vi "Drop Down VI Loader.vi"(7 "Software Config File Path":path=path "C:/Users/Ries Lab/Documents/Microscope Control from Sheng Account/Microscope-Control/Drop Down VI Loader/Drop Down VI Loader Config Files/EMBL 4Pi.txt") -> ()   [LabVIEW 2021]
uses:
  Drop Down VI Loader Type Defs/DDVL Drop Down Bar.ctl
  <vilib>/Utility/miscctls.llb/LVPointTypeDef.ctl
  <vilib>/Utility/miscctls.llb/LVRectTypeDef.ctl
panel:
  in  "Drop Down Control 20":T1
  in  "Drop Down Control 19":T1
  in  "Drop Down Control 18":T1
  in  "Drop Down Control 17":T1
  in  "Drop Down Control 16":T1
  in  "Drop Down Control 15":T1
  in  "Drop Down Control 14":T1
  in  "Drop Down Control 13":T1
  in  "Drop Down Control 12":T1
  in  "Drop Down Control 11":T1
  in  "Hide Exit Bar":bool
  in  "Hide Drop Bars":bool
  in  "Screen and Exit Bar":T2
  in  "Drop Down Control 01":T1
  in  "Drop Down Control 02":T1
  in  "Drop Down Control 03":T1
  in  "Drop Down Control 04":T1
  in  "Drop Down Control 05":T1
  in  "Drop Down Control 06":T1
  in  "Drop Down Control 07":T1
  in  "Drop Down Control 08":T1
  in  "Drop Down Control 09":T1
  in  "Drop Down Control 10":T1
  # "Some Text"
  # "Some Text"
  # "Some Text"
  # "Some Text"
  # "Some Text"
  # "Some Text"
  # "Some Text"
  # "Some Text"
  # "Some Text"
  # "Some Text"
  # "Blank 01"
  # "Blank 02"
  # "Blank 03"
  # "Blank 04"
  # "Blank 05"
  # "Blank 06"
  # "Blank 07"
  # "Blank 08"
  # "Some Text"
  # "Some Text"
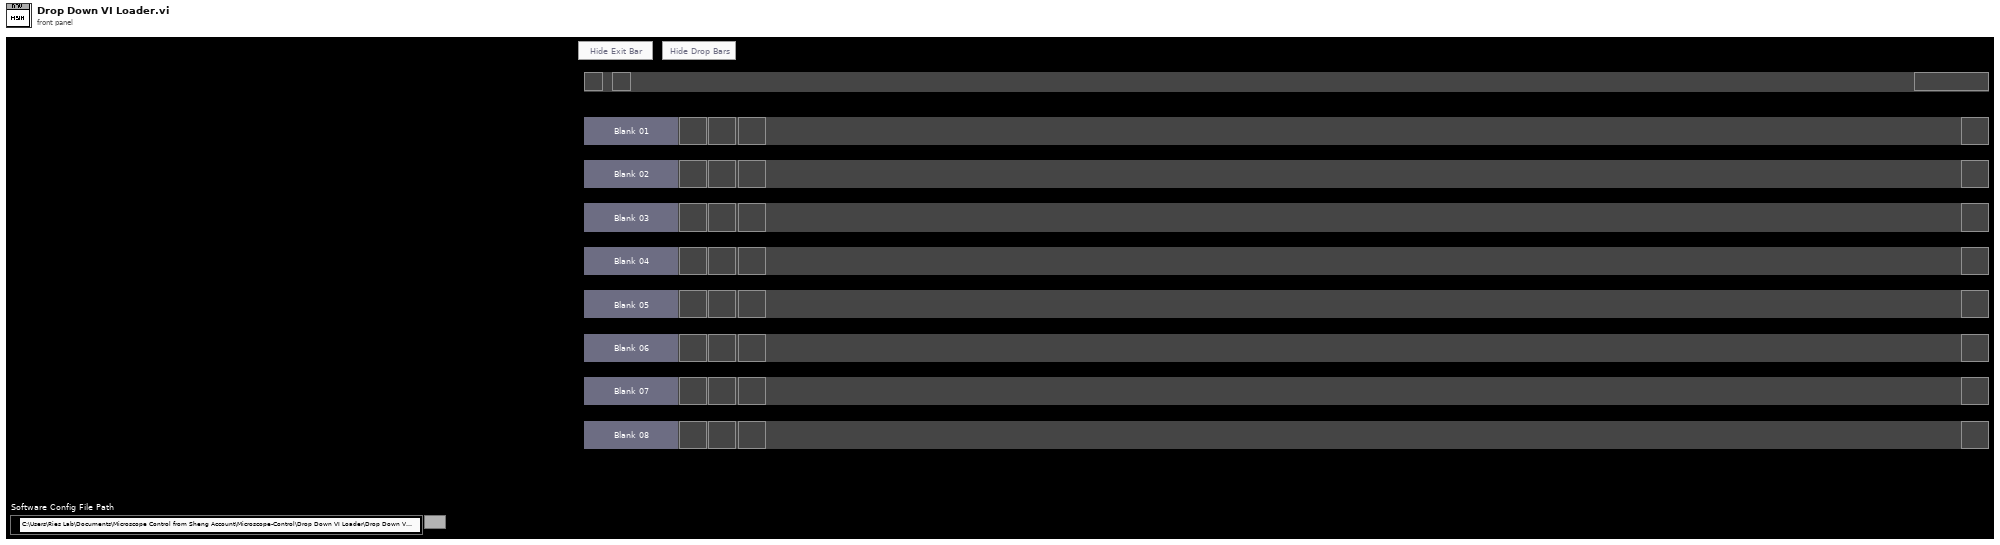
[diagram p1: front panel]
types:
  T1 = typedef "DDVL Drop Down Bar.ctl" = cluster{"Right Width":bool, "Messages":string, "Abort VI":bool, "Close VI":bool, "Pop Out":bool}
  T2 = cluster{"Max Left":bool, "Max Right":bool, "Exit":bool, "Messages":string}
  T3 = enum16{"Always On", "Always Off", "Off While Running"}
  T4 = typedef "LVPointTypeDef.ctl" = cluster{"Horizontal":i16, "Vertical":i16}
  T5 = enum32{"Invalid", "Standard", "Closed", "Hidden", "Minimized", "Maximized"}
  T6 = typedef "LVRectTypeDef.ctl" = cluster{"Left":i16, "Top":i16, "Right":i16, "Bottom":i16}
  T7 = enum8{"Enabled", "Disabled", "Disabled and Grayed Out"}
  T8 = cluster{"VI Path":path, "VI Refnum":refnum<vi>}[]
  T9 = typedef "lveventtype.ctl" = enum32{"Null", "Timeout", "Annotation Menu Selection", "Annotation Menu Selection?", "App Instance Close", "App Instance Close?", "Autoscale Range Change", "Bookmark Info Change", "Cell Edit", "Cell Edit?", "Cursor Grab", "Cursor Grab?", "Cursor Menu Selection", "Cursor Menu Selection?", "Cursor Move", "Cursor Release", "Data Change", "Direction Change", "Display State Change", "Drag Ended", "Drag Enter", "Drag Leave", "Drag Over", "Drag Source Update", "Drag Starting", "Drag Starting?", "Drop", "Exec State Change", "Key Down", "Key Down?", "Key Repeat", "Key Repeat?", "Key Up", "Listbox Double Click", "Menu Activation?", "Menu Selection (App)", "Menu Selection? (App)", "Menu Selection (User)", "Mouse Down", "Mouse Down?", "Mouse Enter", "Mouse Leave", "Mouse Move", "Mouse Up", "Mouse Wheel", "NI Security User Change (App)", "Pane Size", "Panel Close", "Panel Close?", "Panel Resize", "Plot Attribute Change", "Scale Range Change", "Shortcut Menu Activation?", "Shortcut Menu Selection (App)", "Shortcut Menu Selection? (App)", "Shortcut Menu Selection (User)", "Tree Double Click", "Tree Drag", "Tree Drag?", "Tree Drop", "Tree Drop?", "Tree Item Close", "Tree Item Close?", "Tree Item Open", "Tree Item Open?", "User Event", "Value Change"}
  T10 = typedef "LVAllMonitorsDisplayTypeDef.ctl" = cluster{"Bounds":cluster{"Left":i16, "Top":i16, "Right":i16, "Bottom":i16}, "Depth":i16}[]
  T11 = cluster{"Bounds":cluster{"Left":i16, "Top":i16, "Right":i16, "Bottom":i16}, "Depth":i16}
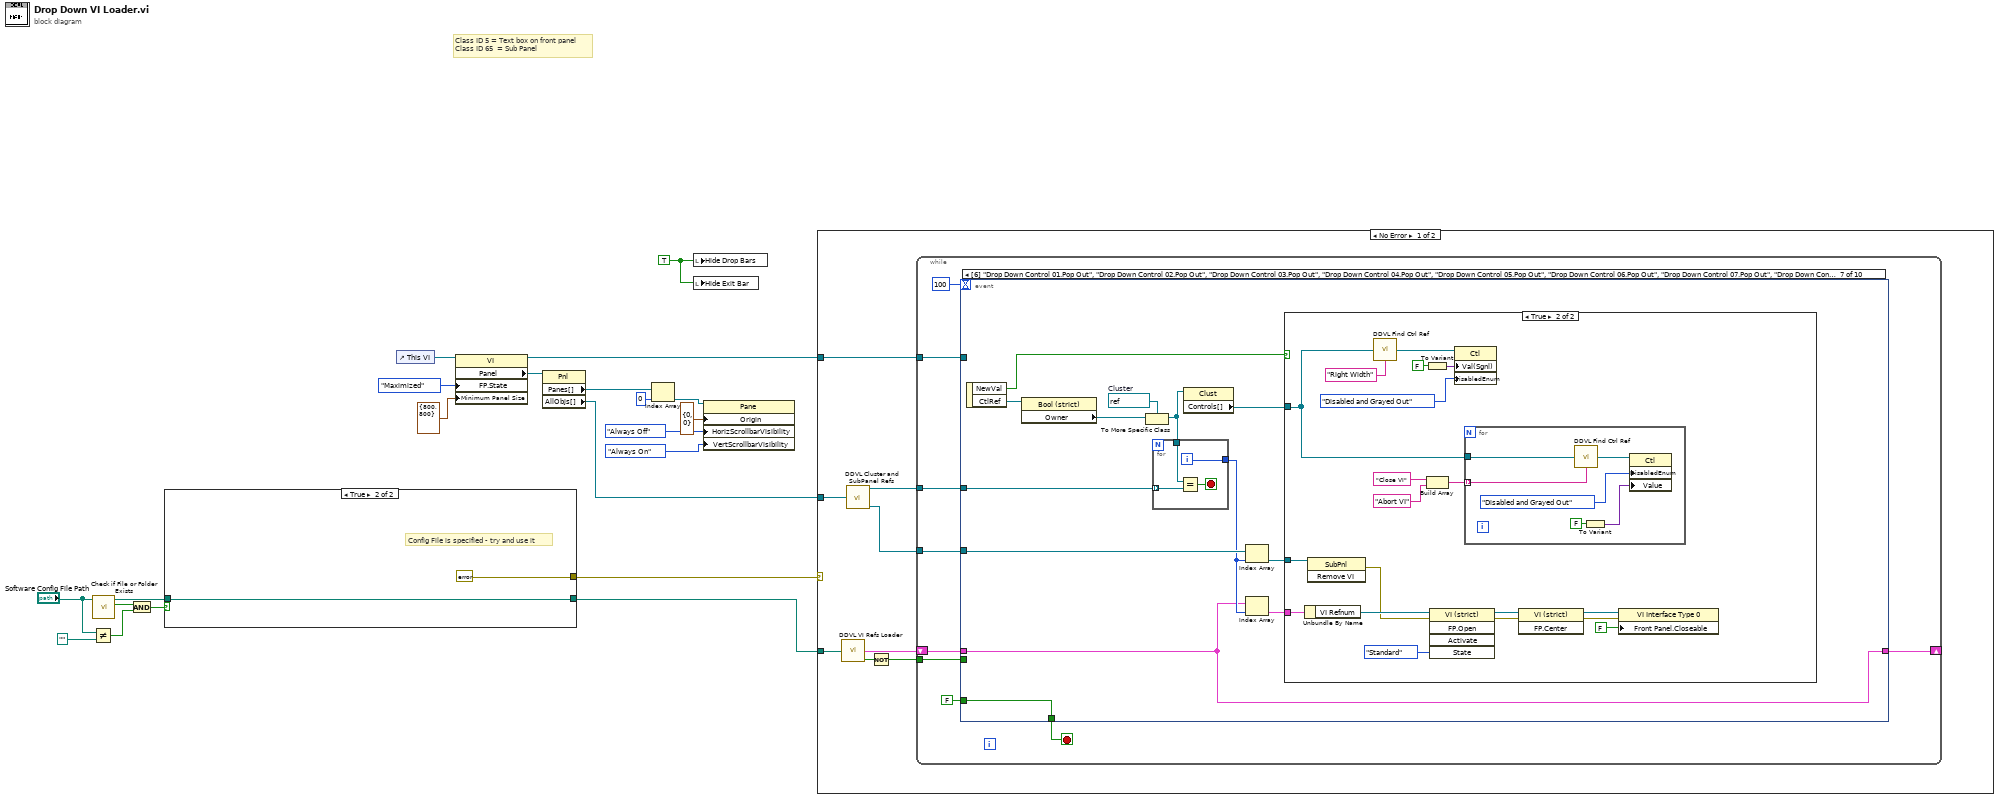
[diagram p0: block diagram]
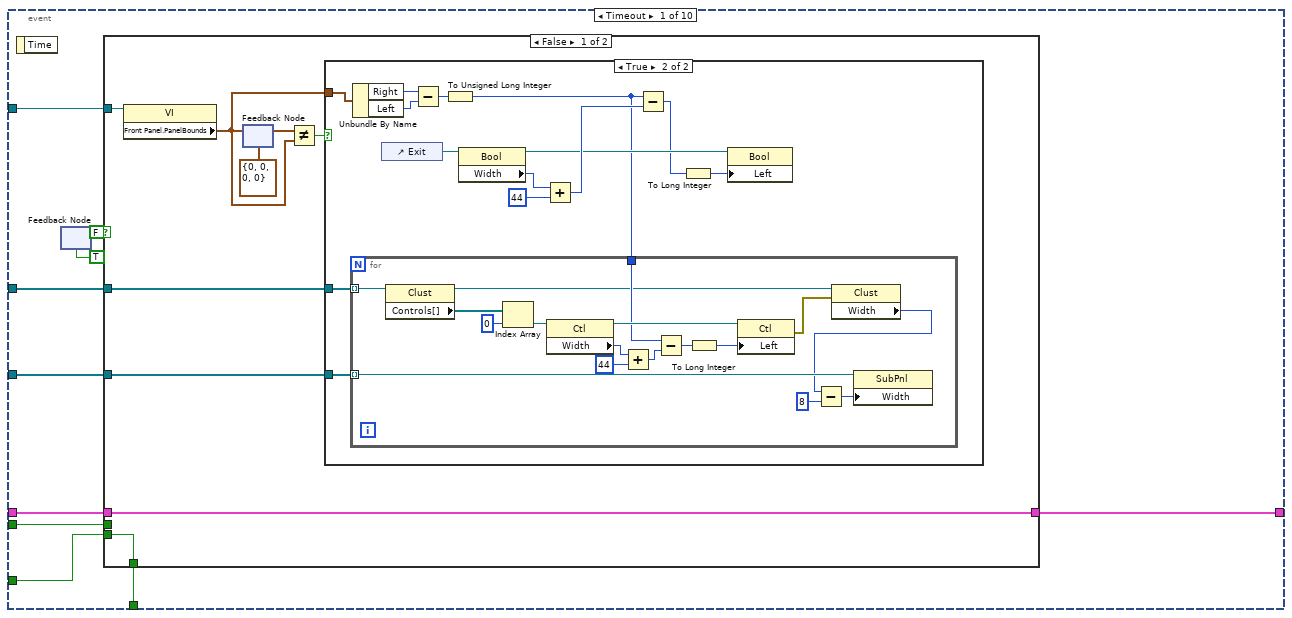
[diagram p2: hidden frame]
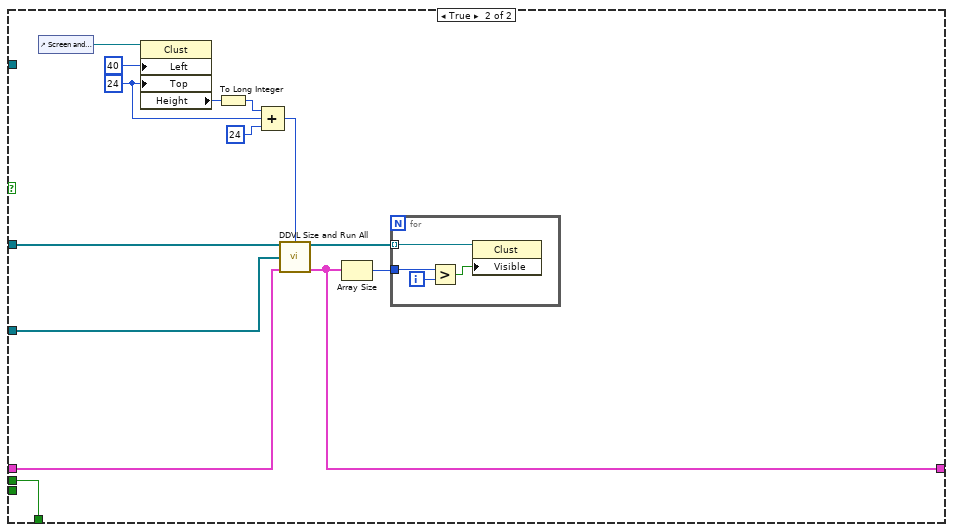
[diagram p4: hidden frame]
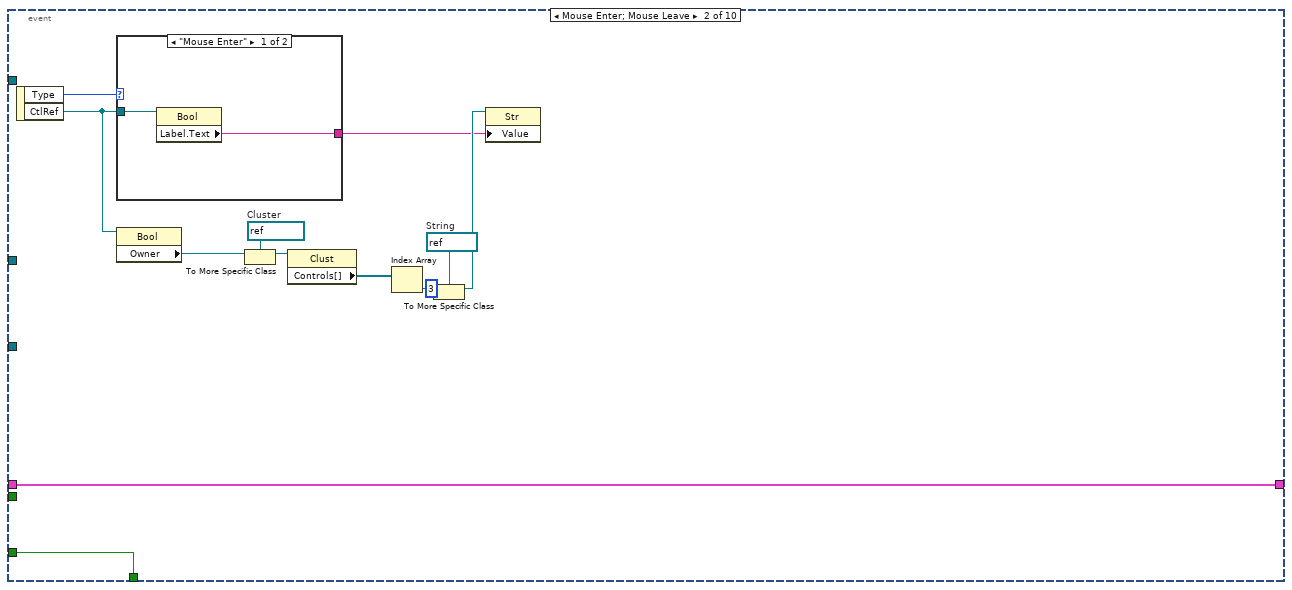
[diagram p5: hidden frame]
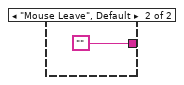
[diagram p6: hidden frame]
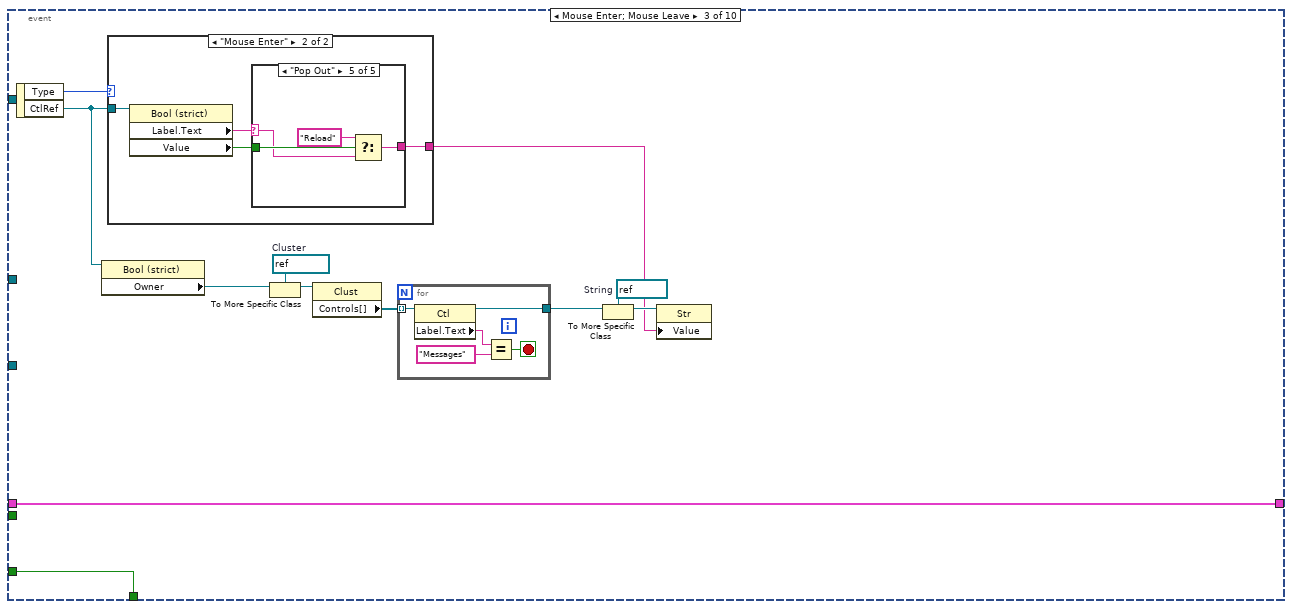
[diagram p7: hidden frame]
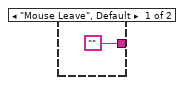
[diagram p8: hidden frame]
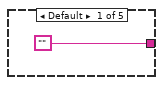
[diagram p9: hidden frame]
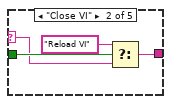
[diagram p10: hidden frame]
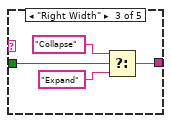
[diagram p11: hidden frame]
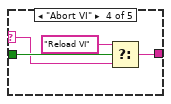
[diagram p12: hidden frame]
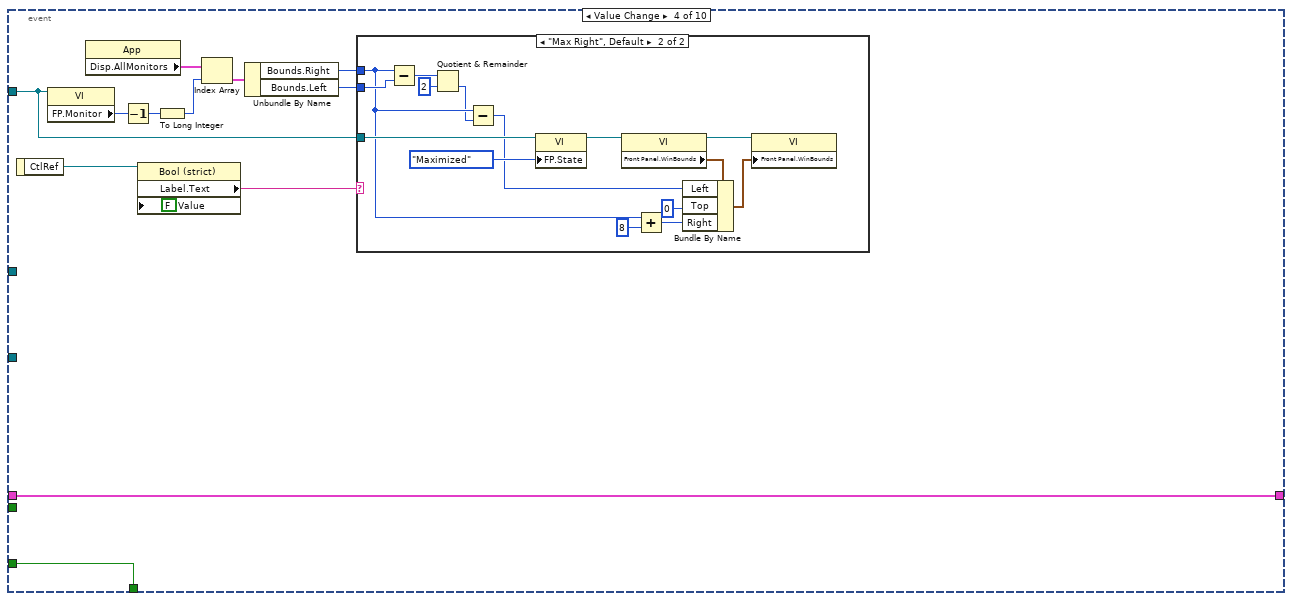
[diagram p13: hidden frame]
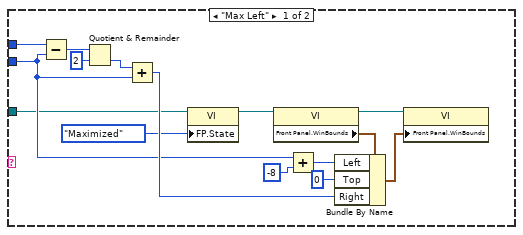
[diagram p14: hidden frame]
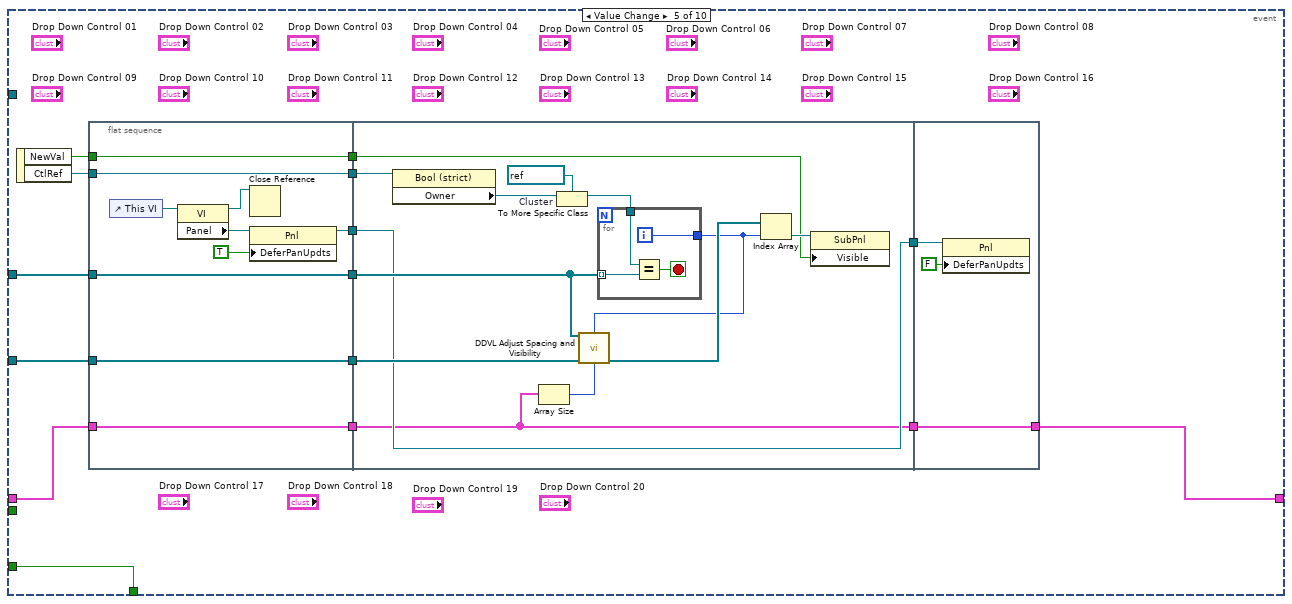
[diagram p15: hidden frame]
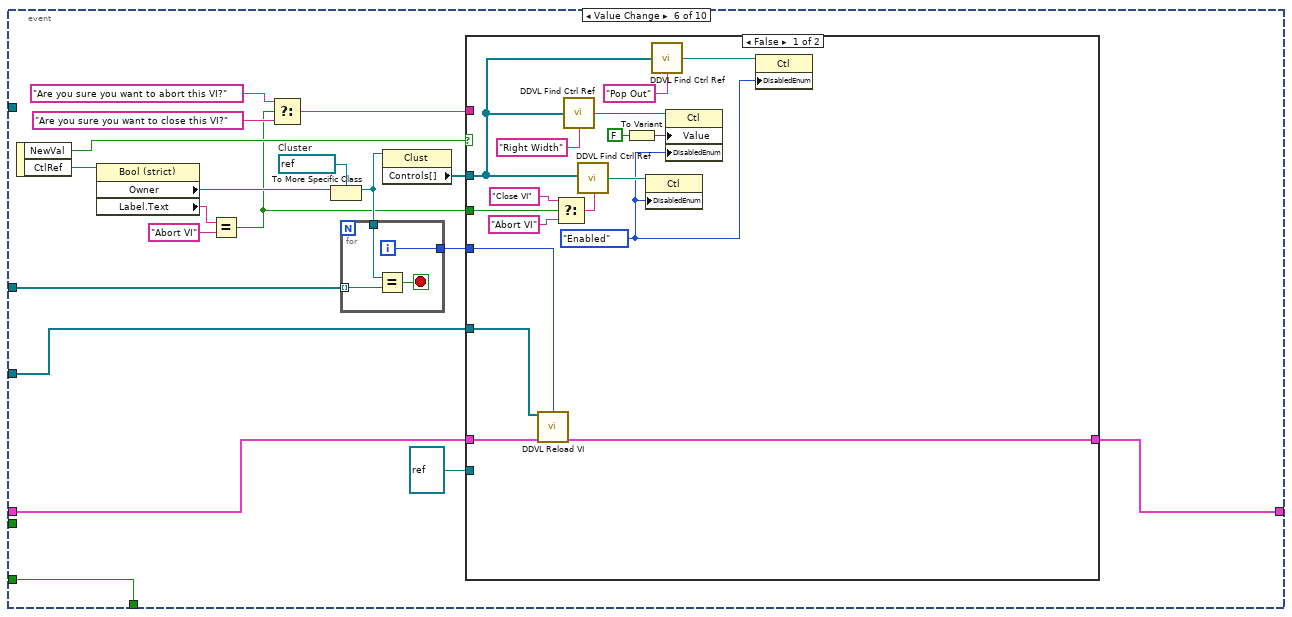
[diagram p16: hidden frame]
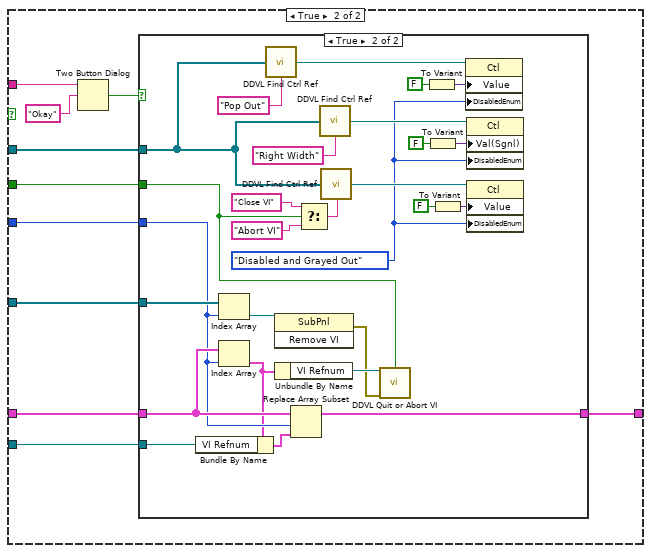
[diagram p17: hidden frame]
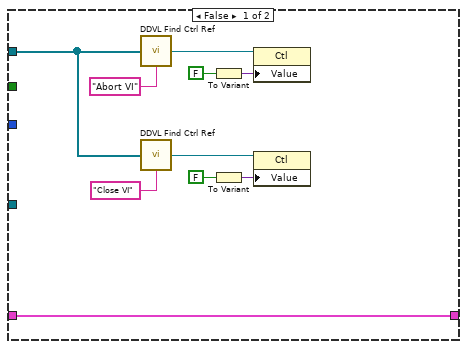
[diagram p18: hidden frame]
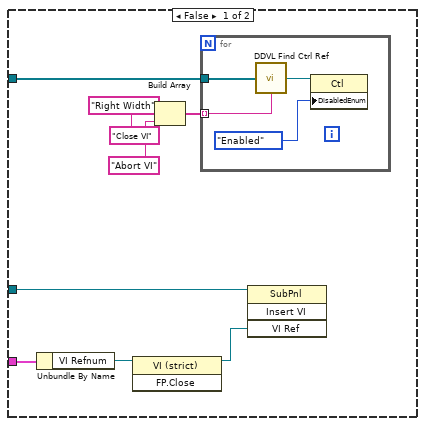
[diagram p19: hidden frame]
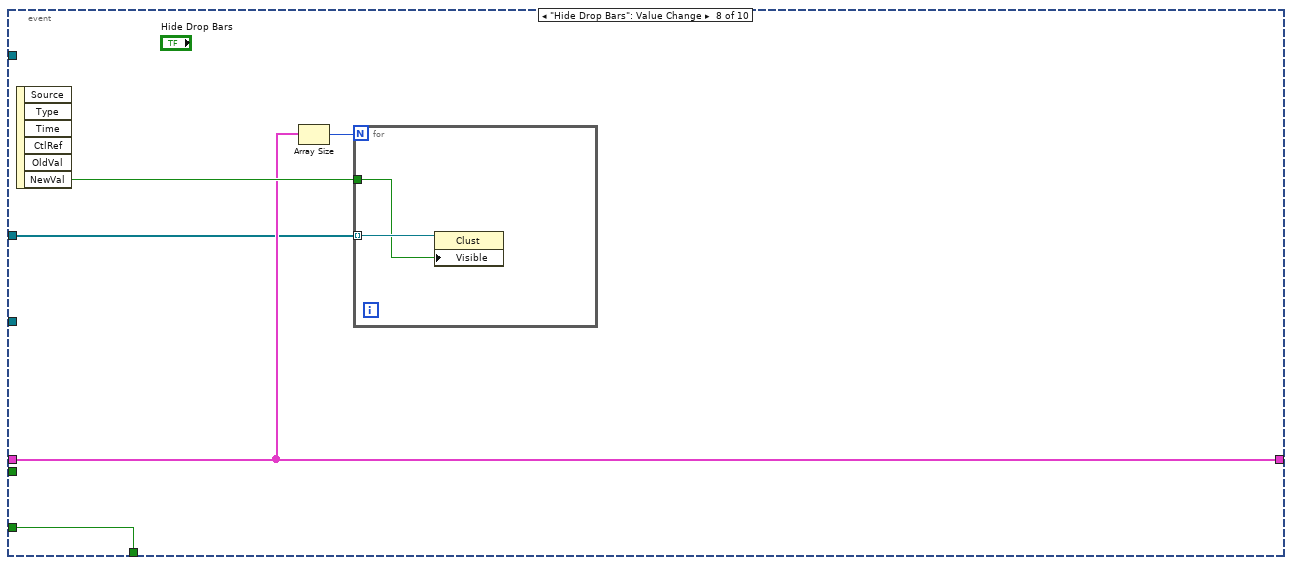
[diagram p20: hidden frame]
diagram:
  w1 = TRUE ("Hide Drop Bars")
  # "Class ID 5 = Text box on front panel\nClass ID 65  = Sub Panel"
  n1 = Not Equal?(x="Software Config File Path", y=path "") -> (x != y?=w8:bool)
  n2 = call <vilib>:"Check if File or Folder Exists.vi"("path"="Software Config File Path") -> ("file or folder exists?"=w7:bool, "dup path"=w5:path)  [unwired: 8 in, 1 out]
  n3 = And(x=w7, y=w8) -> (x .and. y?=w6:bool)
  n4 = case shown="True" w6 {
    tunnel: w5 -> [_ w34]
    tunnel: [w30 w34] -> w2
    tunnel: [w29 errorcluster {"status"=FALSE, "code"=0, "source"=""} ("error out")] -> w3
    frame False {
      # "User must select config file"
      n5 = control-ref of="This VI"() -> (w24:refnum<vi>)
      n6 = property class="VI"(reference=w24) -> ("Path"=w23:path)  [unwired: 1 in, 2 out]
      n7 = Strip Path(path=w23) -> (stripped path=w25:path)  [unwired: 1 out]
      n8 = Path To String(path=w25) -> (string=w26:string)
      n9 = Concatenate Strings(w26, "\\Drop Down VI Loader Config Files") -> (w28:string)
      n10 = String To Path(string=w28) -> (path=w22:path)
      n11 = call "File Dialog"("start path"=w22, "prompt"="Select Software Config File", "pattern (all files)"="*.txt") -> ("selected path"=w30:path, "error out"=w29:errorcluster)  [unwired: 9 in, 2 out]
    }
    frame True {
      # "Config File is specified - try and use it"
    }
  }
  n12 = control-ref of="This VI"() -> (w17:refnum<vi>)
  n13 = property class="VI"(reference=w17, "FP.State"=T5."Maximized" ("Front Panel Window:State"), "Minimum Panel Size"=T4 {"Horizontal"=800, "Vertical"=800} ("Front Panel Window:Minimum Size")) -> (reference out=w12:refnum<vi>, "Panel"=w11:refnum<vi>)  [unwired: 1 in, 1 out]
  n14 = property class="Pnl"(reference=w11) -> ("Panes[]"=w14:refnum<vi>[], "AllObjs[]"=w10:refnum<vi>[])  [unwired: 1 in, 2 out]
  n15 = Index Array(array=w14, index=0) -> (element=w20:refnum<vi>)
  n16 = local write "Hide Drop Bars"(w1) -> ()
  n17 = local write "Hide Exit Bar"(w1) -> ()
  n18 = property class="Pane"(reference=w20, "Origin"=T4 {"Horizontal"=0, "Vertical"=0}, "HorizScrollbarVisibility"=T3."Always Off" ("Vertical Scrollbar Visibility"), "VertScrollbarVisibility"=T3."Always On" ("Vertical Scrollbar Visibility")) -> ()  [unwired: 1 in, 2 out]
  n19 = case shown="No Error" w3 {
    tunnel: w12 -> [w42 _]
    tunnel: w10 -> [w40 _]
    tunnel: w2 -> [w37 _]
    frame No Error {
      n20 = call "DDVL VI Refs Loader.vi"("Config File Path"=w37) -> ("VI Path/Ref"=w39:T8, "VIs Loaded?"=w41:bool)  [unwired: 12 in, 1 out]
      n21 = call "DDVL Cluster and SubPanel Refs.vi"("All Objects Refs"=w40) -> ("Cluster Refs"=w36:refnum<vi>[], "Sub Panel Refs"=w35:refnum<vi>[])  [unwired: 13 in]
      n22 = Not(x=w41) -> (.not. x?=w38:bool)
      n23 = while {
        tunnel: w42 -> [w48]
        tunnel: w36 -> [w43]
        tunnel: w35 -> [w46]
        tunnel: w38 -> [w45]
        shift-right: [w44] -> _
        shift-left: w39 -> [w47]
        stop <- w51 stop-if-true
        n24 = event shown="[6] \"Drop Down Control 01.Pop Out\", \"Drop Down Control 02.Pop Out\", \"Drop Down Control 03.Pop Out\", \"Drop Down Control 04.Pop Out\", \"Drop Down Control 05.Pop Out\", \"Drop Down Control 06.Pop Out\", \"Drop Down Control 07.Pop Out\", \"Drop Down Control 08.Pop Out\", \"Drop Down Control 09.Pop Out\", \"Drop Down Control 10.Pop Out\", \"Drop Down Control 11.Pop Out\", \"Drop Down Control 12.Pop Out\", \"Drop Down Control 13.Pop Out\", \"Drop Down Control 14.Pop Out\", \"Drop Down Control 15.Pop Out\", \"Drop Down Control 16.Pop Out\", \"Drop Down Control 17.Pop Out\", \"Drop Down Control 18.Pop Out\", \"Drop Down Control 19.Pop Out\", \"Drop Down Control 20.Pop Out\": Value Change" {
          selector: _ -> [_ _ _ _ _ _ _ _ _ _]
          dyn-events: _ -> [_ _ _ _ _ _ _ _ _ _]
          timeout: 100 -> [_ _ _ _ _ _ _ _ _ _]
          tunnel: [w58 w133 w147 w188 w233 w282 w363 w410 w416 w432] -> w51
          tunnel: FALSE -> [w57 w133 w147 w188 w233 w282 w363 w410 w416 _]
          tunnel: w48 -> [w62 _ _ w179 _ _ _ _ _ _]
          tunnel: w43 -> [w61 _ _ _ w231 w277 w357 w406 _ w430]
          tunnel: w46 -> [w60 _ _ _ w232 w275 w356 _ _ w429]
          tunnel: w47 -> [w59 w121 w148 w176 w228 w276 w352 w407 w415 w428]
          tunnel: w45 -> [w56 _ _ _ _ _ _ _ _ _]
          tunnel: [w55 w121 w148 w176 w220 w273 w352 w407 w415 w427] -> w44
          event Timeout {
            n25 = event-data() -> ()  [unwired: 1 in, 1 out]
            n26 = feedback #1(TRUE) -> (w52:bool)
            n27 = feedback-in #1(FALSE) -> ()
            n28 = case shown="False" w52 {
              tunnel: w62 -> [w71 _]
              tunnel: w61 -> [w66 w107]
              tunnel: w60 -> [w65 w114]
              tunnel: w59 -> [w63 w113]
              tunnel: [w64 w104] -> w58
              tunnel: w57 -> [w64 _]
              tunnel: w56 -> [_ w104]
              tunnel: [w63 w103] -> w55
              frame False {
                n29 = property class="VI"(reference=w71) -> ("Front Panel.PanelBounds"=w67:T6)  [unwired: 1 in, 2 out]
                n30 = feedback-in #2(w67) -> ()
                n31 = feedback #2(T6 {"Left"=0, "Top"=0, "Right"=0, "Bottom"=0} ("Front Panel.PanelBounds")) -> (w70:T6)
                n32 = Not Equal?(x=w70, y=w67) -> (x != y?=w68:bool)
                n33 = case shown="True" w68 {
                  tunnel: w67 -> [_ w85]
                  tunnel: w66 -> [_ w75]
                  tunnel: w65 -> [_ w72]
                  frame False {
                  }
                  frame True {
                    n34 = Unbundle By Name(w85) -> ("Right"=w77:i16, "Left"=w78:i16)
                    n35 = control-ref of="Exit"() -> (w83:refnum<vi>)
                    n36 = Subtract(x=w77, y=w78) -> (x-y=w76:i16)
                    n37 = To Unsigned Long Integer(number=w76) -> (unsigned 32bit integer=w73:u32)
                    n38 = for {
                      tunnel: w75 -> [w102] mode=indexing
                      tunnel: w73 -> [w93]
                      tunnel: w72 -> [w91] mode=indexing
                      n39 = property class="Clust"(reference=w102) -> (reference out=w90:refnum<vi>, "Controls[]"=w101:refnum<vi>[])  [unwired: 1 in, 1 out]
                      n40 = Index Array(array=w101, index=0) -> (element=w97:refnum<vi>)
                      n41 = property class="Ctl"(reference=w97) -> (reference out=w96:refnum<vi>, "Width"=w98:u32)  [unwired: 1 in, 1 out]
                      n42 = Add(x=w98, y=u32 44) -> (x+y=w95:u32)
                      n43 = Subtract(x=w93, y=w95) -> (x-y=w94:u32)
                      n44 = To Long Integer(number=w94) -> (32bit integer=w99:i32)
                      n45 = property class="Ctl"(reference=w96, "Left"=w99) -> (error out=w89:errorcluster)  [unwired: 1 in, 1 out]
                      n46 = property class="Clust"(reference=w90, error in=w89) -> ("Width"=w88:u32)  [unwired: 2 out]
                      n47 = Subtract(x=w88, y=u32 8) -> (x-y=w87:u32)
                      n48 = property class="SubPnl"(reference=w91, "Width"=w87) -> ()  [unwired: 1 in, 2 out]
                    }
                    n49 = property class="Bool"(reference=w83) -> (reference out=w81:refnum<vi>, "Width"=w84:u32)  [unwired: 1 in, 1 out]
                    n50 = Add(x=w84, y=u32 44) -> (x+y=w82:u32)
                    n51 = Subtract(x=w73, y=w82) -> (x-y=w79:u32)
                    n52 = To Long Integer(number=w79) -> (32bit integer=w80:i32)
                    n53 = property class="Bool"(reference=w81, "Left"=w80) -> ()  [unwired: 1 in, 2 out]
                  }
                }
              }
              frame True {
                w111 = 24 ("Position:Top")
                n54 = control-ref of="Screen and Exit Bar"() -> (w116:refnum<vi>)
                n55 = property class="Clust"(reference=w116, "Left"=40 ("Position:Left"), "Top"=w111) -> ("Height"=w112:u32)  [unwired: 1 in, 2 out]
                n56 = To Long Integer(number=w112) -> (32bit integer=w110:i32)
                n57 = Compound Arithmetic op=ADD(w110, w111, 24 ("value")) -> (w108:i32)
                n58 = call "DDVL Size and Run All.vi"("Cluster Refs"=w107, "Initial Top Position"=w108, "Subpanel Refs"=w114, "VI Path/Ref"=w113) -> ("Cluster Refs Dup"=w106:refnum<vi>[], "VI Path/Ref Out"=w103:T8)  [unwired: 10 in]
                n59 = Array Size(array=w103) -> (size(s)=w105:i32)
                n60 = for {
                  tunnel: w106 -> [w120] mode=indexing
                  tunnel: w105 -> [w117]
                  i -> [w119]
                  n61 = Greater?(x=w117, y=w119) -> (0:w118:bool)
                  n62 = property class="Clust"(reference=w120, "Visible"=w118) -> ()  [unwired: 1 in, 2 out]
                }
              }
            }
          }
          event "Screen and Exit Bar.Exit", "Screen and Exit Bar.Max Right", "Screen and Exit Bar.Max Left": Mouse Enter; "Screen and Exit Bar.Exit", "Screen and Exit Bar.Max Right", "Screen and Exit Bar.Max Left": Mouse Leave {
            w124 = refnum<vi> refnum  # String
            w129 = refnum<vi> refnum  # Cluster
            n63 = event-data() -> ("Type"=w132:T9, "CtlRef"=w131:refnum<vi>)  [unwired: 1 in]
            n64 = case shown="\"Mouse Enter\"" w132 {
              tunnel: w131 -> [w135 _]
              tunnel: [w134 ""] -> w122
              frame "Mouse Enter" {
                n65 = property class="Bool"(reference=w135) -> ("Label.Text"=w134:string)  [unwired: 1 in, 2 out]
              }
              frame "Mouse Leave", Default {
              }
            }
            n66 = property class="Bool"(reference=w131) -> ("Owner"=w130:refnum<vi>)  [unwired: 1 in, 2 out]
            n67 = To More Specific Class(target class=w129, reference=w130) -> (specific class reference=w128:refnum<vi>)  [unwired: 1 in, 1 out]
            n68 = property class="Clust"(reference=w128) -> ("Controls[]"=w127:refnum<vi>[])  [unwired: 1 in, 2 out]
            n69 = Index Array(array=w127, index=3) -> (element=w125:refnum<vi>)
            n70 = To More Specific Class(target class=w124, reference=w125) -> (specific class reference=w123:refnum<vi>)  [unwired: 1 in, 1 out]
            n71 = property class="Str"(reference=w123, "Value"=w122) -> ()  [unwired: 1 in, 2 out]
          }
          event Mouse Enter; Mouse Leave {
            w139 = refnum<vi> refnum  # String
            w144 = refnum<vi> refnum  # Cluster
            n72 = event-data() -> ("Type"=w146:T9, "CtlRef"=w145:refnum<vi>)  [unwired: 1 in]
            n73 = property class="Bool (strict)"(reference=w145) -> ("Owner"=w142:refnum<vi>)  [unwired: 1 in, 2 out]
            n74 = case shown="\"Mouse Enter\"" w146 {
              tunnel: w145 -> [_ w158]
              tunnel: ["" w155] -> w137
              frame "Mouse Leave", Default {
              }
              frame "Mouse Enter" {
                n75 = property class="Bool (strict)"(reference=w158) -> ("Label.Text"=w157:string, "Value"=w156:bool)  [unwired: 1 in, 2 out]
                n76 = case shown="\"Pop Out\"" w157 {
                  selector: w157 -> [_ w162 _ w169 w173]
                  tunnel: w156 -> [_ w163 w167 w170 w174]
                  tunnel: ["" w160 w164 w168 w172] -> w155
                  frame Default {
                  }
                  frame "Close VI" {
                    n77 = Select(t="Reload VI", s=w163, f=w162) -> (s? t:f=w160:string)
                  }
                  frame "Right Width" {
                    n78 = Select(t="Collapse", s=w167, f="Expand") -> (s? t:f=w164:string)
                  }
                  frame "Abort VI" {
                    n79 = Select(t="Reload VI", s=w170, f=w169) -> (s? t:f=w168:string)
                  }
                  frame "Pop Out" {
                    n80 = Select(t="Reload", s=w174, f=w173) -> (s? t:f=w172:string)
                  }
                }
              }
            }
            n81 = To More Specific Class(target class=w144, reference=w142) -> (specific class reference=w143:refnum<vi>)  [unwired: 1 in, 1 out]
            n82 = property class="Clust"(reference=w143) -> ("Controls[]"=w141:refnum<vi>[])  [unwired: 1 in, 2 out]
            n83 = for {
              tunnel: w141 -> [w153] mode=indexing
              tunnel: [w149] -> w140
              stop <- w150 stop-if-true
              n84 = property class="Ctl"(reference=w153) -> (reference out=w149:refnum<vi>, "Label.Text"=w152:string)  [unwired: 1 in, 1 out]
              n85 = Equal?(x=w152, y="Messages") -> (x = y?=w150:bool)
            }
            n86 = To More Specific Class(target class=w139, reference=w140) -> (specific class reference=w138:refnum<vi>)  [unwired: 1 in, 1 out]
            n87 = property class="Str"(reference=w138, "Value"=w137) -> ()  [unwired: 1 in, 2 out]
          }
          event "Screen and Exit Bar.Max Right", "Screen and Exit Bar.Max Left": Value Change {
            n88 = event-data() -> ("CtlRef"=w187:refnum<vi>)  [unwired: 1 in]
            n89 = property class="VI"(reference=w179) -> ("FP.Monitor"=w186:u16)  [unwired: 1 in, 2 out]
            n90 = property class="App"() -> ("Disp.AllMonitors"=w185:T10)  [unwired: 2 in, 2 out]
            n91 = Decrement(x=w186) -> (x-1=w184:u16)
            n92 = property class="Bool (strict)"(reference=w187, "Value"=FALSE) -> ("Label.Text"=w178:string)  [unwired: 1 in, 2 out]
            n93 = To Long Integer(number=w184) -> (32bit integer=w183:i32)
            n94 = Index Array(array=w185, index=w183) -> (element=w182:T11)
            n95 = Unbundle By Name(w182) -> ("Bounds.Right"=w181:i16, "Bounds.Left"=w180:i16)
            n96 = case shown="\"Max Right\", Default" w178 {
              tunnel: w181 -> [w203 w206]
              tunnel: w180 -> [w191 w210]
              tunnel: w179 -> [w189 w209]
              frame "Max Left" {
                n97 = Subtract(x=w203, y=w191) -> (x-y=w198:i16)
                n98 = Quotient & Remainder(x=w198, y=i16 2) -> (floor(x/y)=w196:i16)  [unwired: 1 out]
                n99 = Add(x=w196, y=w191) -> (x+y=w195:i16)
                n100 = property class="VI"(reference=w189, "FP.State"=T5."Maximized" ("Front Panel Window:State")) -> (reference out=w193:refnum<vi>)  [unwired: 1 in, 1 out]
                n101 = property class="VI"(reference=w193) -> (reference out=w202:refnum<vi>, "Front Panel.WinBounds"=w200:T6)  [unwired: 1 in, 1 out]
                n102 = Add(x=w191, y=i16 -8 ("Left")) -> (x+y=w190:i16)
                n103 = Bundle By Name(cluster=w200, "Left"=w190, "Top"=i16 0, "Right"=w195) -> (w201:T6)
                n104 = property class="VI"(reference=w202, "Front Panel.WinBounds"=w201) -> ()  [unwired: 1 in, 2 out]
              }
              frame "Max Right", Default {
                n105 = Subtract(x=w206, y=w210) -> (x-y=w215:i16)
                n106 = Quotient & Remainder(x=w215, y=i16 2) -> (floor(x/y)=w205:i16)  [unwired: 1 out]
                n107 = Subtract(x=w206, y=w205) -> (x-y=w204:i16)
                n108 = property class="VI"(reference=w209, "FP.State"=T5."Maximized" ("Front Panel Window:State")) -> (reference out=w212:refnum<vi>)  [unwired: 1 in, 1 out]
                n109 = property class="VI"(reference=w212) -> (reference out=w218:refnum<vi>, "Front Panel.WinBounds"=w216:T6)  [unwired: 1 in, 1 out]
                n110 = Add(x=w206, y=i16 8 ("Left")) -> (x+y=w207:i16)
                n111 = Bundle By Name(cluster=w216, "Left"=w204, "Top"=i16 0, "Right"=w207) -> (w217:T6)
                n112 = property class="VI"(reference=w218, "Front Panel.WinBounds"=w217) -> ()  [unwired: 1 in, 2 out]
              }
            }
          }
          event Value Change {
            n113 = event-data() -> ("NewVal"=w229:bool, "CtlRef"=w230:refnum<vi>)  [unwired: 1 in]
            n114 = flat-sequence {
              tunnel: w228 -> [w239]
              tunnel: w229 -> [w240]
              tunnel: w230 -> [w241]
              tunnel: w231 -> [w242]
              tunnel: w232 -> [w243]
              tunnel: [w243] -> w227
              tunnel: [w242] -> w226
              tunnel: [w241] -> w225
              tunnel: [w240] -> w224
              tunnel: [w239] -> w223
              tunnel: [w234] -> w221
              tunnel: w227 -> [w254]
              tunnel: w226 -> [w253]
              tunnel: w225 -> [w252]
              tunnel: w224 -> [w248]
              tunnel: w223 -> [w244]
              tunnel: [w245] -> w222
              tunnel: w221 -> [w245]
              tunnel: [w244] -> w219
              tunnel: w222 -> [w263]
              tunnel: [w261] -> w220
              tunnel: w219 -> [w261]
              frame #0 {
                n115 = control-ref of="This VI"() -> (w236:refnum<vi>)
                n116 = property class="VI"(reference=w236) -> (reference out=w235:refnum<vi>, "Panel"=w237:refnum<vi>)  [unwired: 1 in, 1 out]
                n117 = Close Reference(reference=w235) -> ()  [unwired: 1 in, 1 out]
                n118 = property class="Pnl"(reference=w237, "DeferPanUpdts"=TRUE ("Defer Panel Updates")) -> (reference out=w234:refnum<vi>)  [unwired: 1 in, 1 out]
              }
              frame #1 {
                w250 = refnum<vi> refnum  # Cluster
                n119 = property class="Bool (strict)"(reference=w252) -> ("Owner"=w251:refnum<vi>)  [unwired: 1 in, 2 out]
                n120 = Array Size(array=w244) -> (size(s)=w246:i32)
                n121 = To More Specific Class(target class=w250, reference=w251) -> (specific class reference=w249:refnum<vi>)  [unwired: 1 in, 1 out]
                n122 = for {
                  tunnel: w253 -> [w260] mode=indexing
                  tunnel: w249 -> [w259]
                  tunnel: [w257] -> w247
                  i -> [w257]
                  stop <- w258 stop-if-true
                  n123 = Equal?(x=w259, y=w260) -> (x = y?=w258:bool)
                }
                n124 = call "DDVL Adjust Spacing and Visibility.vi"("Cluster Ref Array"=w253, "Position Index"=w247, "Sub Panel Ref Array"=w254, "Num of VIs"=w246) -> ("Sub Panel Ref Array Dup"=w256:refnum<vi>[])  [unwired: 11 in]
                n125 = Index Array(array=w256, index=w247) -> (element=w255:refnum<vi>)
                n126 = property class="SubPnl"(reference=w255, "Visible"=w248) -> ()  [unwired: 1 in, 2 out]
              }
              frame #2 {
                n127 = property class="Pnl"(reference=w263, "DeferPanUpdts"=FALSE ("Defer Panel Updates")) -> ()  [unwired: 1 in, 2 out]
              }
            }
          }
          event Value Change {
            w280 = refnum<vi> refnum  # Cluster
            n128 = event-data() -> ("NewVal"=w274:bool, "CtlRef"=w279:refnum<vi>)  [unwired: 1 in]
            n129 = property class="Bool (strict)"(reference=w279) -> ("Owner"=w281:refnum<vi>, "Label.Text"=w271:string)  [unwired: 1 in, 2 out]
            n130 = Equal?(x=w271, y="Abort VI" ("message")) -> (x = y?=w264:bool)
            n131 = Select(t="Are you sure you want to abort this VI?" ("message"), s=w264, f="Are you sure you want to close this VI?" ("message")) -> (s? t:f=w267:string)
            n132 = To More Specific Class(target class=w280, reference=w281) -> (specific class reference=w266:refnum<vi>)  [unwired: 1 in, 1 out]
            n133 = for {
              tunnel: w277 -> [w350] mode=indexing
              tunnel: w266 -> [w349]
              tunnel: [w347] -> w278
              i -> [w347]
              stop <- w348 stop-if-true
              n134 = Equal?(x=w349, y=w350) -> (x = y?=w348:bool)
            }
            n135 = property class="Clust"(reference=w266) -> ("Controls[]"=w265:refnum<vi>[])  [unwired: 1 in, 2 out]
            n136 = case shown="False" w274 {
              tunnel: w278 -> [w296 w307]
              tunnel: w276 -> [w298 w306]
              tunnel: w275 -> [w299 w305]
              tunnel: w265 -> [w285 w301]
              tunnel: [w297 w304] -> w273
              tunnel: refnum<vi> refnum ("VI Refnum") -> [_ w303]
              tunnel: w267 -> [_ w302]
              tunnel: w264 -> [w292 w300]
              frame False {
                w283 = T7."Enabled" ("Disabled")
                n137 = call "DDVL Reload VI.vi"("Sub Panel Refs"=w299, "Index"=w296, "Path/Ref Array In"=w298) -> ("Updated Path/Ref Array"=w297:T8)  [unwired: 12 in]
                n138 = Select(t="Close VI" ("message"), s=w292, f="Abort VI" ("message")) -> (s? t:f=w293:string)
                n139 = call "DDVL Find Ctrl Ref.vi"("Control Array"=w285, "Control Label"="Right Width") -> ("Control Ref"=w289:refnum<vi>)  [unwired: 12 in, 1 out]
                n140 = call "DDVL Find Ctrl Ref.vi"("Control Array"=w285, "Control Label"=w293) -> ("Control Ref"=w291:refnum<vi>)  [unwired: 12 in, 1 out]
                n141 = To Variant(anything=FALSE) -> (Variant=w287:variant)
                n142 = property class="Ctl"(reference=w291, "DisabledEnum"=w283) -> ()  [unwired: 1 in, 2 out]
                n143 = call "DDVL Find Ctrl Ref.vi"("Control Array"=w285, "Control Label"="Pop Out") -> ("Control Ref"=w284:refnum<vi>)  [unwired: 12 in, 1 out]
                n144 = property class="Ctl"(reference=w289, "Value"=w287, "DisabledEnum"=w283) -> ()  [unwired: 1 in, 2 out]
                n145 = property class="Ctl"(reference=w284, "DisabledEnum"=w283) -> ()  [unwired: 1 in, 2 out]
              }
              frame True {
                n146 = Two Button Dialog(message=w302, 2:"Okay" ("T button name (\"OK\")")) -> (T button?=w308:bool)  [unwired: 1 in]
                n147 = case shown="True" w308 {
                  tunnel: w307 -> [_ w341]
                  tunnel: w305 -> [_ w346]
                  tunnel: w306 -> [w319 w342]
                  tunnel: [w319 w339] -> w304
                  tunnel: w303 -> [_ w338]
                  tunnel: w301 -> [w313 w322]
                  tunnel: w300 -> [_ w331]
                  frame False {
                    n148 = call "DDVL Find Ctrl Ref.vi"("Control Array"=w313, "Control Label"="Abort VI") -> ("Control Ref"=w314:refnum<vi>)  [unwired: 12 in, 1 out]
                    n149 = call "DDVL Find Ctrl Ref.vi"("Control Array"=w313, "Control Label"="Close VI") -> ("Control Ref"=w312:refnum<vi>)  [unwired: 12 in, 1 out]
                    n150 = To Variant(anything=FALSE) -> (Variant=w317:variant)
                    n151 = To Variant(anything=FALSE) -> (Variant=w316:variant)
                    n152 = property class="Ctl"(reference=w314, "Value"=w317) -> ()  [unwired: 1 in, 2 out]
                    n153 = property class="Ctl"(reference=w312, "Value"=w316) -> ()  [unwired: 1 in, 2 out]
                  }
                  frame True {
                    w320 = T7."Disabled and Grayed Out" ("Disabled")
                    n154 = Index Array(array=w346, index=w341) -> (element=w345:refnum<vi>)
                    n155 = Index Array(array=w342, index=w341) -> (element=w337:cluster{"VI Path":path, "VI Refnum":refnum<vi>})
                    n156 = Bundle By Name(cluster=w337, "VI Refnum"=w338) -> (w340:cluster{"VI Path":path, "VI Refnum":refnum<vi>})
                    n157 = call "DDVL Find Ctrl Ref.vi"("Control Array"=w322, "Control Label"="Pop Out") -> ("Control Ref"=w321:refnum<vi>)  [unwired: 12 in, 1 out]
                    n158 = invoke class="SubPnl" method="Remove VI"(reference=w345) -> (error out=w332:errorcluster)  [unwired: 2 in, 2 out]
                    n159 = Unbundle By Name(w337) -> ("VI Refnum"=w333:refnum<vi>)
                    n160 = Replace Array Subset(array=w342, new element=w340, index=w341) -> (w339:T8)
                    n161 = Select(t="Close VI" ("message"), s=w331, f="Abort VI" ("message")) -> (s? t:f=w334:string)
                    n162 = call "DDVL Find Ctrl Ref.vi"("Control Array"=w322, "Control Label"="Right Width") -> ("Control Ref"=w329:refnum<vi>)  [unwired: 12 in, 1 out]
                    n163 = call "DDVL Find Ctrl Ref.vi"("Control Array"=w322, "Control Label"=w334) -> ("Control Ref"=w326:refnum<vi>)  [unwired: 12 in, 1 out]
                    n164 = call "DDVL Quit or Abort VI.vi"("VI Ref"=w333, "Abort VI?"=w331, "Error In"=w332) -> ()  [unwired: 12 in, 1 out]
                    n165 = To Variant(anything=FALSE) -> (Variant=w324:variant)
                    n166 = To Variant(anything=FALSE) -> (Variant=w327:variant)
                    n167 = To Variant(anything=FALSE) -> (Variant=w344:variant)
                    n168 = property class="Ctl"(reference=w321, "Value"=w324, "DisabledEnum"=w320) -> ()  [unwired: 1 in, 2 out]
                    n169 = property class="Ctl"(reference=w329, "Val(Sgnl)"=w327, "DisabledEnum"=w320) -> ()  [unwired: 1 in, 2 out]
                    n170 = property class="Ctl"(reference=w326, "Value"=w344, "DisabledEnum"=w320) -> ()  [unwired: 1 in, 2 out]
                  }
                }
              }
            }
          }
          event Value Change {
            w361 = refnum<vi> refnum  # Cluster
            n171 = event-data() -> ("NewVal"=w358:bool, "CtlRef"=w359:refnum<vi>)  [unwired: 1 in]
            n172 = property class="Bool (strict)"(reference=w359) -> ("Owner"=w362:refnum<vi>)  [unwired: 1 in, 2 out]
            n173 = To More Specific Class(target class=w361, reference=w362) -> (specific class reference=w360:refnum<vi>)  [unwired: 1 in, 1 out]
            n174 = for {
              tunnel: w357 -> [w364] mode=indexing
              tunnel: w360 -> [w367]
              tunnel: [w365] -> w354
              i -> [w365]
              stop <- w366 stop-if-true
              n175 = Equal?(x=w367, y=w364) -> (x = y?=w366:bool)
            }
            n176 = property class="Clust"(reference=w360) -> ("Controls[]"=w351:refnum<vi>[])  [unwired: 1 in, 2 out]
            n177 = Index Array(array=w356, index=w354) -> (element=w355:refnum<vi>)
            n178 = Index Array(array=w352, index=w354) -> (element=w353:cluster{"VI Path":path, "VI Refnum":refnum<vi>})
            n179 = case shown="True" w358 {
              tunnel: w355 -> [w375 w399]
              tunnel: w353 -> [w376 w398]
              tunnel: w351 -> [w372 w384]
              frame False {
                n180 = Unbundle By Name(w376) -> ("VI Refnum"=w374:refnum<vi>)
                n181 = invoke class="VI (strict)" method="FP.Close"(reference=w374) -> (reference out=w373:refnum<vi>)  [unwired: 2 in, 2 out]
                n182 = Build Array("Right Width" ("Control Label"), "Close VI" ("message"), "Abort VI" ("message")) -> (w368:string[])
                n183 = for {
                  tunnel: w372 -> [w378]
                  tunnel: w368 -> [w377] mode=indexing
                  n184 = call "DDVL Find Ctrl Ref.vi"("Control Array"=w378, "Control Label"=w377) -> ("Control Ref"=w380:refnum<vi>)  [unwired: 12 in, 1 out]
                  n185 = property class="Ctl"(reference=w380, "DisabledEnum"=T7."Enabled" ("Disabled")) -> ()  [unwired: 1 in, 2 out]
                }
                n186 = invoke class="SubPnl" method="Insert VI"(reference=w375, "VI Ref"=w373) -> ()  [unwired: 2 in, 4 out]
              }
              frame True {
                n187 = Unbundle By Name(w398) -> ("VI Refnum"=w397:refnum<vi>)
                n188 = invoke class="SubPnl" method="Remove VI"(reference=w399) -> (error out=w393:errorcluster)  [unwired: 2 in, 2 out]
                n189 = call "DDVL Find Ctrl Ref.vi"("Control Array"=w384, "Control Label"="Right Width") -> ("Control Ref"=w391:refnum<vi>)  [unwired: 12 in, 1 out]
                n190 = To Variant(anything=FALSE) -> (Variant=w389:variant)
                n191 = Build Array("Close VI" ("message"), "Abort VI" ("message")) -> (w385:string[])
                n192 = invoke class="VI (strict)" method="FP.Open"(reference=w397, error in=w393, "State"=T5."Standard") -> (reference out=w395:refnum<vi>, error out=w394:errorcluster)  [unwired: 2 in, 3 out]
                n193 = property class="Ctl"(reference=w391, "Val(Sgnl)"=w389, "DisabledEnum"=T7."Disabled and Grayed Out" ("Disabled")) -> ()  [unwired: 1 in, 2 out]
                n194 = for {
                  tunnel: w384 -> [w403]
                  tunnel: w385 -> [w402] mode=indexing
                  n195 = call "DDVL Find Ctrl Ref.vi"("Control Array"=w403, "Control Label"=w402) -> ("Control Ref"=w405:refnum<vi>)  [unwired: 12 in, 1 out]
                  n196 = To Variant(anything=FALSE) -> (Variant=w400:variant)
                  n197 = property class="Ctl"(reference=w405, "DisabledEnum"=T7."Disabled and Grayed Out" ("Disabled"), "Value"=w400) -> ()  [unwired: 1 in, 2 out]
                }
                n198 = invoke class="VI (strict)" method="FP.Center"(reference=w395, error in=w394) -> (reference out=w383:refnum<vi>, error out=w381:errorcluster)  [unwired: 1 in, 1 out]
                n199 = property class="VI Interface Type 0"(reference=w383, error in=w381, "Front Panel.Closeable"=FALSE ("Front Panel Window:Closeable")) -> ()  [unwired: 2 out]
              }
            }
          }
          event "Hide Drop Bars": Value Change {
            n200 = event-data() -> ("NewVal"=w409:bool)  [unwired: 1 in, 5 out]
            n201 = Array Size(array=w407) -> (size(s)=w408:i32)
            n202 = for {
              N: w408 -> [_]
              tunnel: w406 -> [w412] mode=indexing
              tunnel: w409 -> [w411]
              n203 = property class="Clust"(reference=w412, "Visible"=w411) -> ()  [unwired: 1 in, 2 out]
            }
          }
          event "Hide Exit Bar": Value Change {
            n204 = event-data() -> ("NewVal"=w413:bool)  [unwired: 1 in]
            n205 = control-ref of="Screen and Exit Bar"() -> (w414:refnum<vi>)
            n206 = property class="Clust"(reference=w414, "Visible"=w413) -> ()  [unwired: 1 in, 2 out]
          }
          event "Screen and Exit Bar.Exit": Value Change {
            n207 = event-data() -> ("NewVal"=w432:bool)  [unwired: 1 in]
            n208 = property on="Messages" class="Str"("Value"="") -> ()  [unwired: 2 in, 2 out]
            n209 = flat-sequence {
              tunnel: w429 -> [w443]
              tunnel: w430 -> [w444]
              tunnel: [w444] -> w421
              tunnel: [w443] -> w420
              tunnel: [w434] -> w419
              tunnel: [w433] -> w417
              tunnel: w421 -> [w448]
              tunnel: w420 -> [w447]
              tunnel: w419 -> [w446]
              tunnel: [w445] -> w418
              tunnel: w417 -> [w445]
              tunnel: w418 -> [w468]
              frame #0 {
                n210 = control-ref of="Screen and Exit Bar"() -> (w437:refnum<vi>)
                n211 = control-ref of="This VI"() -> (w440:refnum<vi>)
                n212 = property class="VI"(reference=w440) -> (reference out=w439:refnum<vi>, "Panel"=w441:refnum<vi>)  [unwired: 1 in, 1 out]
                n213 = property class="Clust"(reference=w437) -> ("Height"=w438:u32)  [unwired: 1 in, 2 out]
                n214 = Close Reference(reference=w439) -> ()  [unwired: 1 in, 1 out]
                n215 = property class="Pnl"(reference=w441, "DeferPanUpdts"=TRUE ("Defer Panel Updates")) -> (reference out=w433:refnum<vi>)  [unwired: 1 in, 1 out]
                n216 = To Long Integer(number=w438) -> (32bit integer=w436:i32)
                n217 = Add(x=w436, y=48) -> (x+y=w434:i32)
              }
              frame #1 {
                n218 = for {
                  tunnel: w448 -> [w457] mode=indexing
                  shift-right: [w456] -> _
                  shift-left: w446 -> [w452]
                  tunnel: w447 -> [w449] mode=indexing
                  n219 = property class="SubPnl"(reference=w449, "Visible"=FALSE) -> ()  [unwired: 1 in, 2 out]
                  n220 = property class="Clust"(reference=w457, "Left"=40 ("Position:Left"), "Top"=w452) -> ("Controls[]"=w451:refnum<vi>[], "Height"=w454:u32)  [unwired: 1 in, 2 out]
                  n221 = To Long Integer(number=w454) -> (32bit integer=w453:i32)
                  n222 = for {
                    tunnel: w451 -> [w463] mode=indexing
                    n223 = property class="Ctl"(reference=w463) -> (reference out=w459:refnum<vi>, "ClassID"=w462:u32)  [unwired: 1 in, 1 out]
                    n224 = Equal?(x=w462, y=u32 8) -> (x = y?=w460:bool)
                    n225 = case shown="True" w460 {
                      tunnel: w459 -> [_ w465]
                      frame False {
                      }
                      frame True {
                        n226 = To Variant(anything=FALSE) -> (Variant=w466:variant)
                        n227 = property class="Ctl"(reference=w465, "Value"=w466, "DisabledEnum"=T7."Enabled" ("Disabled")) -> ()  [unwired: 1 in, 2 out]
                      }
                    }
                  }
                  n228 = Compound Arithmetic op=ADD(w453, w452, 12 ("value")) -> (w456:i32)
                }
              }
              frame #2 {
                n229 = property class="Pnl"(reference=w468, "DeferPanUpdts"=FALSE ("Defer Panel Updates")) -> ()  [unwired: 1 in, 2 out]
              }
            }
            n230 = for {
              tunnel: w428 -> [w478] mode=indexing
              tunnel: [w478] -> w427 mode=indexing
              shift-right: [w472] -> w422
              shift-left: "The following VIs could not be\nclosed successfully:\n" -> [w473]
              tunnel: [w471] -> w425 mode=indexing
              n231 = Unbundle By Name(w478) -> ("VI Path"=w475:path, "VI Refnum"=w477:refnum<vi>)
              n232 = call "DDVL Quit or Abort VI.vi"("VI Ref"=w477, "Abort VI?"=FALSE) -> ("Close Command Successful?"=w471:bool)  [unwired: 13 in]
              n233 = call <vilib>:"Get File Extension.vi"("file"=w475) -> ("filename without extension"=w474:string)  [unwired: 6 in, 4 out]
              n234 = case shown="False" w471 {
                tunnel: w474 -> [w481 _]
                tunnel: w473 -> [w480 w483]
                tunnel: [w479 w483] -> w472
                frame False {
                  n235 = Concatenate Strings(w480, w481, "\r") -> (w479:string)
                }
                frame True {
                }
              }
            }
            n236 = Not(x=w425) -> (.not. x?=w424:bool[])
            n237 = Or Array Elements(Boolean array=w424) -> (logical OR=w423:bool)
            n238 = case shown="True" w423 {
              tunnel: w422 -> [_ w470]
              frame False {
              }
              frame True {
                n239 = One Button Dialog(message=w470) -> ()  [unwired: 1 in, 1 out]
              }
            }
          }
        }
      }
    }
    frame Error {
    }
  }
